vi "Mouse In.vi"(8 "error in (no error)":errorcluster, 10 "MousePoint":cluster{"x":i16, "y":i16}, 11 "Graphic in":refnum<class "Graphic.lvclass">) -> (0 "error out":errorcluster, 2 "In?":bool, 3 "Graphic out":refnum<class "Graphic.lvclass">)   [LabVIEW 2015, in "Graphic.lvclass"]
uses:
  Graphic.lvclass
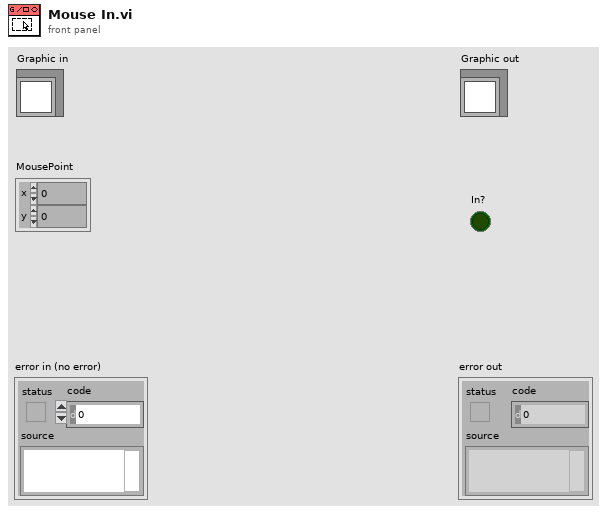
[diagram p1: front panel]
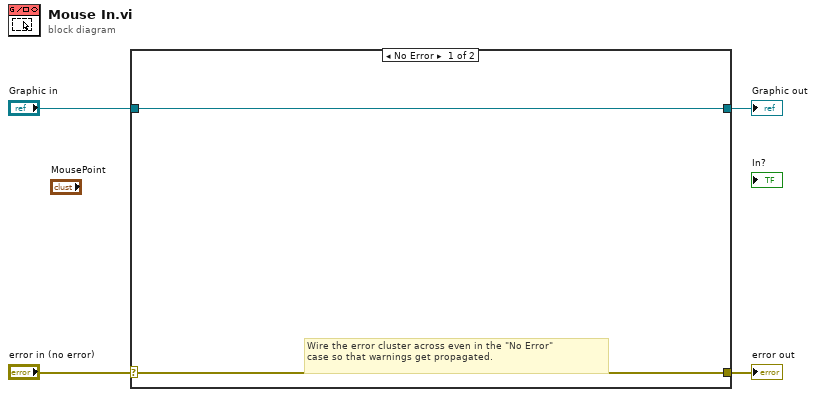
[diagram p0: block diagram]
diagram:
  n1 = case shown="No Error" "error in (no error)" {
    selector: "error in (no error)" -> [w5 w8]
    tunnel: [w5 w8] -> w3
    tunnel: [w6 w7] -> w1
    tunnel: "Graphic in" -> [w6 w7]
    frame No Error {
      # "Wire the error cluster across even in the \"No Error\"\ncase so that warnings get propagated."
    }
    frame Error {
    }
  }
  "error out" <- w3
  "Graphic out" <- w1
